vi "Encoders Reset.vi"(8 "error in (no error)":errorcluster, 11 "TitanENC in":T1) -> (0 "error out":errorcluster, 3 "TitanENC":T2)   [LabVIEW 2020]
uses:
  <vilib>/High Genius/HG_WSI_Tookit/Dependencies/Library/TitanENC/TitanENC.lvclass
  <vilib>/High Genius/HG_WSI_Tookit/Dependencies/Library/VMX Library.lvlib
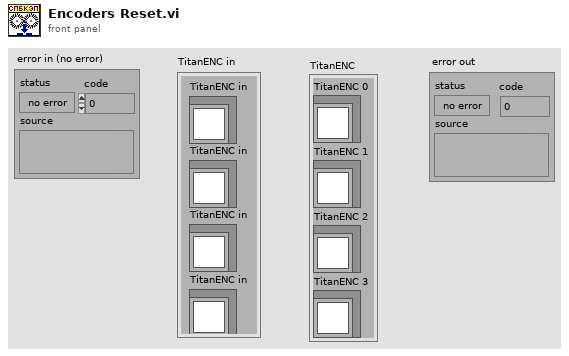
[diagram p1: front panel]
types:
  T1 = cluster{"TitanENC in":refnum<class "TitanENC.lvclass">, "TitanENC in":refnum<class "TitanENC.lvclass">, "TitanENC in":refnum<class "TitanENC.lvclass">, "TitanENC in":refnum<class "TitanENC.lvclass">}
  T2 = cluster{"TitanENC 0":refnum<class "TitanENC.lvclass">, "TitanENC 1":refnum<class "TitanENC.lvclass">, "TitanENC 2":refnum<class "TitanENC.lvclass">, "TitanENC 3":refnum<class "TitanENC.lvclass">}
  T3 = typedef "Semaphore RefNum" = refnum<k1>
  T4 = cluster{"titanenc0":i32, "titanenc1":i32, "titanenc2":i32, "titanenc3":i32, "rpm0":i16, "rpm1":i16, "rpm2":i16, "rpm3":i16, "resetenc0":bool, "resetenc1":bool, "resetenc2":bool, "resetenc3":bool}
  T5 = cluster{"data":cluster{"ai22":sgl, "ai23":sgl, "ai24":sgl, "ai25":sgl, "pulse12":i32, "pulse13":i32, "pwm14":i32, "pwm15":i32, "pwm16":dbl, "do17":bool, "do18":bool, "do19":bool, "do20":bool, "do21":bool, "di11":bool, "di9":bool, "motor0":u8, "motor1":u8, "motor2":u8, "motor3":u8, "dir00":u8, "dir01":u8, "dir02":u8, "dir03":u8, "dir10":u8, "dir11":u8, "dir12":u8, "dir13":u8, "limit0":bool, "limit1":bool, "limit2":bool, "limit3":bool, "limit4":bool, "limit5":bool, "limit6":bool, "limit7":bool, "lsb0H":u8, "lsb1H":u8, "lsb2H":u8, "lsb3H":u8, "lsb0L":u8, "lsb1L":u8, "lsb2L":u8, "lsb3L":u8, "enc0_counters":u32, "enc1_counters":u32, "enc2_counters":u32, "enc3_counters":u32, "counter10":u32, "counter8":u32, "reset_enc0":bool, "reset_enc1":bool, "reset_enc2":bool, "reset_enc3":bool, "pitch":sgl, "roll":sgl, "yaw":sgl, "zero_yaw":bool}}
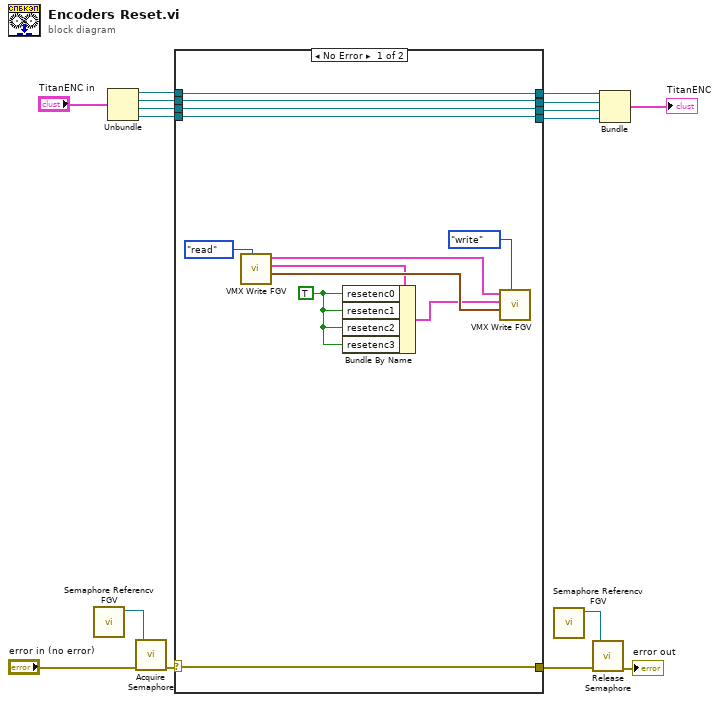
[diagram p0: block diagram]
diagram:
  n1 = call <vilib>:"Semaphore Referencv FGV.vi"() -> ("Semaphore Reference"=w15:T3)  [unwired: 11 in]
  n2 = Unbundle("TitanENC in") -> ("TitanENC in"=w4:refnum<class "TitanENC.lvclass">, "TitanENC in"=w3:refnum<class "TitanENC.lvclass">, "TitanENC in"=w2:refnum<class "TitanENC.lvclass">, "TitanENC in"=w1:refnum<class "TitanENC.lvclass">)
  n3 = call <vilib>:"Acquire Semaphore.vi"("error in (no error)"="error in (no error)", "semaphore"=w15) -> ("error out"=w16:errorcluster)  [unwired: 3 in, 2 out]
  n4 = case shown="No Error" w16 {
    selector: w16 -> [w27 w33]
    tunnel: [w27 w33] -> w13
    tunnel: [w23 w32] -> w8
    tunnel: w4 -> [w23 w32]
    tunnel: [w22 w31] -> w7
    tunnel: [w21 w30] -> w6
    tunnel: [w20 w29] -> w5
    tunnel: w3 -> [w22 w31]
    tunnel: w2 -> [w21 w30]
    tunnel: w1 -> [w20 w29]
    frame No Error {
      w17 = TRUE
      n5 = call <vilib>:"VMX Write FGV.vi"("Enum"=enum16{"read", "write"}."read") -> ("Read Data3"=w24:cluster{"pwm17":i32, "pwm18":i32}, "Read Data2"=w19:T4, "Read Data"=w25:T5)  [unwired: 8 in]
      n6 = Bundle By Name(cluster=w19, "resetenc0"=w17, "resetenc1"=w17, "resetenc2"=w17, "resetenc3"=w17) -> (w18:T4)
      n7 = call <vilib>:"VMX Write FGV.vi"("Enum"=enum16{"read", "write"}."write", "Write Data3"=w24, "Write Data2"=w18, "Write Data"=w25) -> ()  [unwired: 5 in, 3 out]
    }
    frame Error {
    }
  }
  n8 = call <vilib>:"Semaphore Referencv FGV.vi"() -> ("Semaphore Reference"=w14:T3)  [unwired: 11 in]
  n9 = call <vilib>:"Release Semaphore.vi"("error in (no error)"=w13, "semaphore"=w14) -> ("error out"=→"error out":errorcluster)  [unwired: 4 in, 1 out]
  n10 = Bundle("TitanENC in"=w8, "TitanENC in"=w7, "TitanENC in"=w6, "TitanENC in"=w5) -> (→"TitanENC":T1)  [unwired: 1 in]
